vi "Clear Hardware.vi"(2 "error in (no error)":errorcluster, 3 "DDS in":refnum<class "DDS.lvclass"> caption="Device in") -> (0 "error out":errorcluster, 1 "DDS out":refnum<class "DDS.lvclass"> caption="Device out")   [LabVIEW 2013, in "DDS.lvclass"]
doc: "This VI resets any necessary hardware so that the device will be ready for the next run."
uses:
  DDS.lvclass
  Device/Device.lvclass
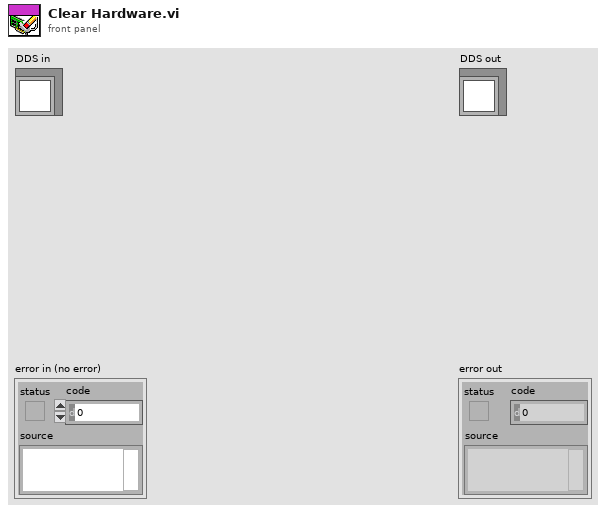
[diagram p1: front panel]
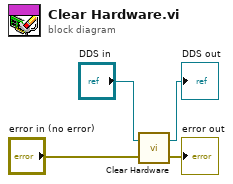
[diagram p0: block diagram]
diagram:
  n1 = call-parent "Clear Hardware.vi"("error in (no error)"="error in (no error)", "Device in"="DDS in") -> ("error out"=→"error out":errorcluster, "Device out"=→"DDS out":refnum<class "DDS.lvclass">)
